vi "BiopsyBatch.vi"() -> ()   [LabVIEW 2022 SP3]
uses:
  <vilib>/Utility/file.llb/Read From Spreadsheet File (DBL).vi
  <vilib>/Analysis/NI_AALBase.lvlib
  <vilib>/Analysis/baseanly.llb/Mean (DBL).vi
panel:
  out "inc x (mm)":dbl format="%.3f"
  out "inc y (mm)":dbl format="%.3f"
  in  "Correct Data?":bool
  in  "RF pts in line":i32=110
  in  "fix rf pts?":bool=TRUE
  in  "Batch file source":u16(ring) items=["Single eye file", "All files in chosen directory", "Choose directroy and file list"]
  out "Current File":string
  in  "Choose Directory of EYE files":path=path "C:/WINDOWS/DESKTOP/rri.eye"
  out "single case fit data":T1 {"pts in fit" format="%.2f"; "midband fit" format="%.2f"; "intercept (b)" format="%.2f"; "slope (m)" format="%.3f"}
  in  "which cursors?":bool
  out "polar axis":cluster{"r axis":dbl[], "theta axis":dbl[]} {"theta axis" format="%.2f"; "r axis" format="%.2f"}
  in  "Log scaling?":bool=TRUE
  out "raw x coord":dbl[][](array[numeric]) format="%.2f"
  out "raw y coord":dbl[][](array[numeric]) format="%.2f"
  out "raw sector image":dbl[][](array[numeric]) format="%.2f"
  out "Axis scaling Params":T2 {"Y high" format="%.2f"; "Y low" format="%.2f"; "X left" format="%.2f"; "X right" format="%.2f"}
  out "Sector as data array":dbl[][](graph)
  in  "Last sector file":path
  in  "View Header?":bool
  in  "Save to Spectra.txt?":bool
  out "Cal File Att":string
  out "RF File Att":string
  in  "FFT size for":u16(ring)=6 items=["next 2^n", "8", "16", "32", "64", "128", "256", "512"]
  in  "Cal File Selection":u16(ring)=1 items=["Don't subtract a Cal File", "Use Info in Header", "Specify Cal Info"]
  in  "Cal File Name":string
  out "actual length\nof padded ROI":i32
  out "need this # of RF pts\nto match Cal File":i32
  in  "Fit band":T3={"start"=3.5, "stop freq"=8.0, "center freq"=5.75} {"center freq" format="%.2f"; "stop freq" format="%.2f"; "start" format="%.2f"}
  out "Spectrum (dBr vs. MHz)":T4(graph)
  out "Raw data":i16[][](graph)
  in  "new eye file path":path
  # "Define endpoints of biopsy ROI. Normally only need to define green and red cursor. Green lower left, red upper left, yellow lower right. Default values are those used in MSKCC study. ROI must be set up with data having 8 mm delay. Run program, then choose a file with 8 mm delay when prompted. Program can then be run again in batch mode by selecting Save to Spectra.txt. Batch operation is done on a whole directory or a list of files. Batch mode will adjust ROI to account for any cases that do not have an 8 mm delay."
  # "Spectrum Fit Parameters"
  # "Only top and bottom of sector box is shown. Ends\nmay not stop at the same scan line."
  # "© 2000-2002 Riverside Research Institute"
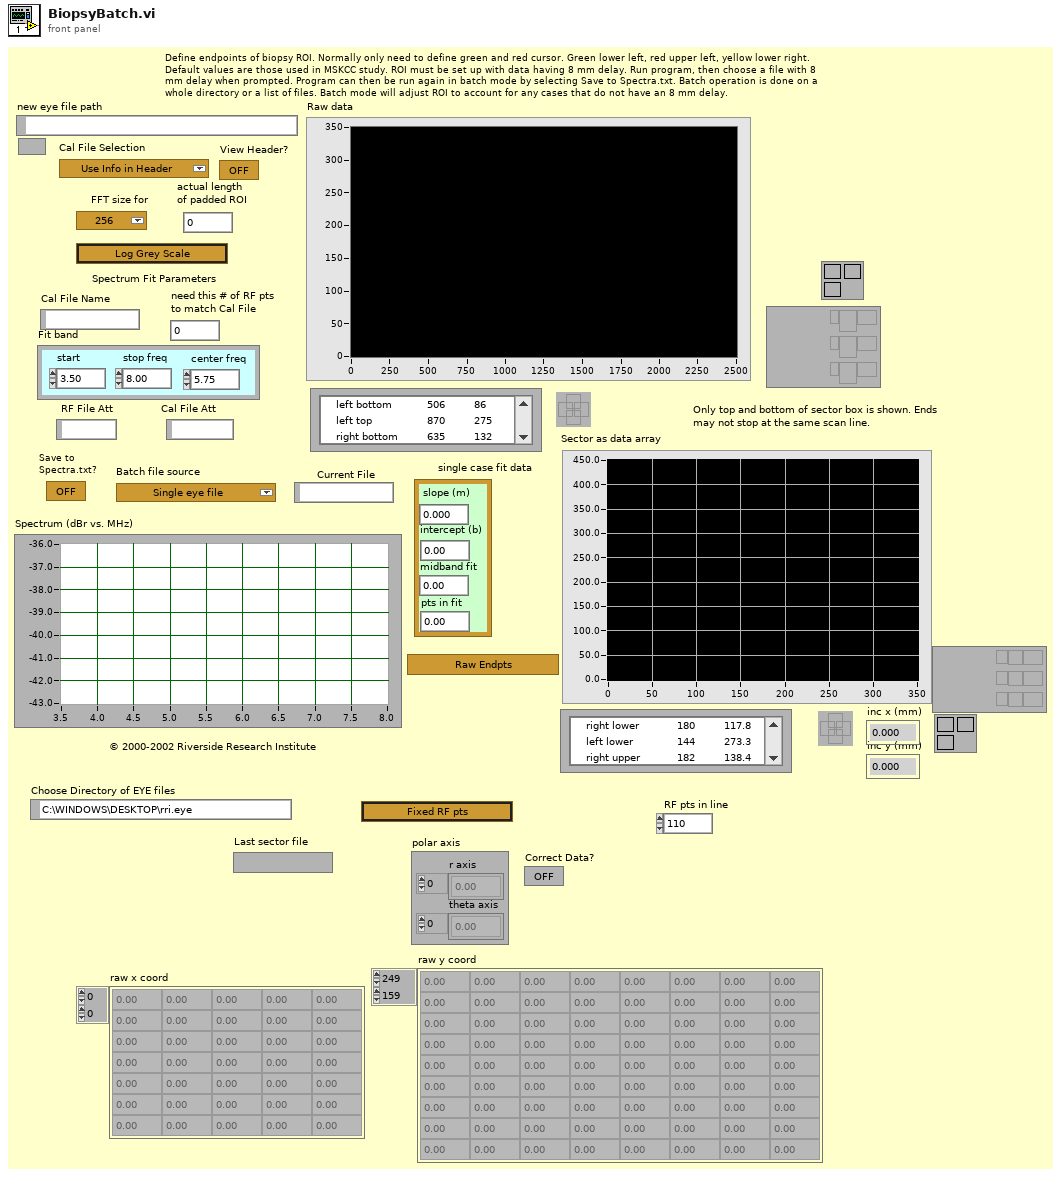
[diagram p1: front panel]
types:
  T1 = cluster{"slope (m)":dbl, "intercept (b)":dbl, "midband fit":dbl, "pts in fit":dbl}
  T2 = cluster{"X right":dbl, "X left":dbl, "Y low":dbl, "Y high":dbl}
  T3 = cluster{"start":dbl, "stop freq":dbl, "center freq":dbl}
  T4 = cluster{"fo of fit":dbl, "df (MHz)":dbl, "Best Linear Fit":dbl[]}[]
  T5 = typedef "Header.ctl" = cluster{"header info":cluster{"Header":string, "Head length":i16}, "A/D info":cluster{"# rf points per line":u16, "# lines per scan":u16, "sample rate MHz":u16, "# A/D bits":i16, "# bytes per A/D":u16, "TGC Flag":u16, "A/D Type":string}, "Tranducer Info":cluster{"bandwidth":sgl, "center freq":sgl, "start freq":sgl, "ID":i32}, "Scan Info":cluster{"delay":sgl, "pivot distance":sgl, "sector scan angle":sgl, "operator":string, "Scan Mode":string, "location":string}, "Time/Date Info":cluster{"date":string, "time":string}, "RF Info":cluster{"RF file name":string, "RF file att":string, "RF cal file name":string, "RF cal file att":string}, "Patient Info":cluster{"ID":string, "extended ID":string, "age":u16, "sex":string, "previously\nscanned":string, "PSA":sgl, "LOS":u8, "Ethnicty 2":u8, "Race":u8}, "Tissue Type":cluster{"organ":i16, "disease type":i16, "disease location":i16, "IQ_pts":u16, "RcvBuffer":u8, "RcvFrame":u16, "IQBuff":u8, "IQFrame":u16, "IQPage":u8}, "Votage scaling":cluster{"Digitizer (dB)":sgl, "Gain (dB)":sgl, "Atten (dB)":sgl}, "Comment":string, "Misc Info":cluster{"avg num":u16, "c speed":i16, "Div By or SF zones":i16, "XMIT CHS":u8, "RCV CHS":u8, "Xmit angle":sgl}, "Therapy Parameters":cluster{"Theraputic Freq (MHz)":sgl, "Time on (s)":sgl, "Therapy amplitude (mV)":sgl, "Lines Before":u16, "Lines After":u16}, "Scan Settings":cluster{"Energy (uJ or V)":u8, "Damp (Ohm) or Fc":u8, "HP Filt (KHz)":u8, "LP Filt (MHz)":u8, "Gain (db)":u8, "prf (kHz)":sgl, "Distance between\nscan lines (um)":u16, "Distance between\nscan planes (um)":u16, "Scan line gap (um)":sgl, "Scan plane gap (um)":sgl}, "Compression Parameters":cluster{"F1 (MHz)":sgl, "F2 (MHz)":sgl, "% taper":sgl, "duration":sgl}, "Patient Info Xtra":cluster{"First Name":string, "Last Name":string, "Notes":string}, "ROI Box":u16[]}
  T6 = cluster{"delay":sgl, "pivot distance":sgl, "sector scan angle":sgl, "operator":string, "Scan Mode":string, "location":string}
  T7 = cluster{"Cursor.Cursor X":dbl, "Cursor.Cursor Y":dbl, "Cursor.Cursor X":dbl, "Cursor.Cursor Y":dbl, "Cursor.Cursor X":dbl, "Cursor.Cursor Y":dbl, i32, i32}
  T8 = enum32{"existing file", "new file", "new or existing file", "existing dir", "new dir", "new or existing dir", "existing file (use LLBs)", "new file (use LLBs)", "new or existing file (use LLBs)", "new or existing file or directory (use LLBs)"}
  T9 = cluster{"bandwidth":sgl, "center freq":sgl, "start freq":sgl, "ID":i32}
  T10 = cluster{"RF file name":string, "RF file att":string, "RF cal file name":string, "RF cal file att":string}
  T11 = cluster{"RF file name":string, "RF file att":string, "Cal File Name":string, "RF cal file att":string}
  T12 = cluster{"start freq":sgl, sgl, "center freq":sgl}
  T13 = cluster{"sample rate MHz":u16, "first row":dbl[], "Fit band":cluster{"start":dbl, "stop freq":dbl, "center freq":dbl}, "RF Info":cluster{"RF file name":string, "RF file att":string, "RF cal file name":string, "RF cal file att":string}, "2-D data array":i16[][], "delay":sgl}
  T14 = cluster{"mean":dbl, "RF pts in line":i32, "Cursor.Cursor Y":dbl, i32}
  T15 = cluster{"slope (m)":dbl[][], "intercept (b)":dbl[][], "midband fit":dbl[][], "pts in fit":dbl}
  T16 = cluster{"fo of fit":dbl, "df (MHz)":dbl, dbl[]}[]
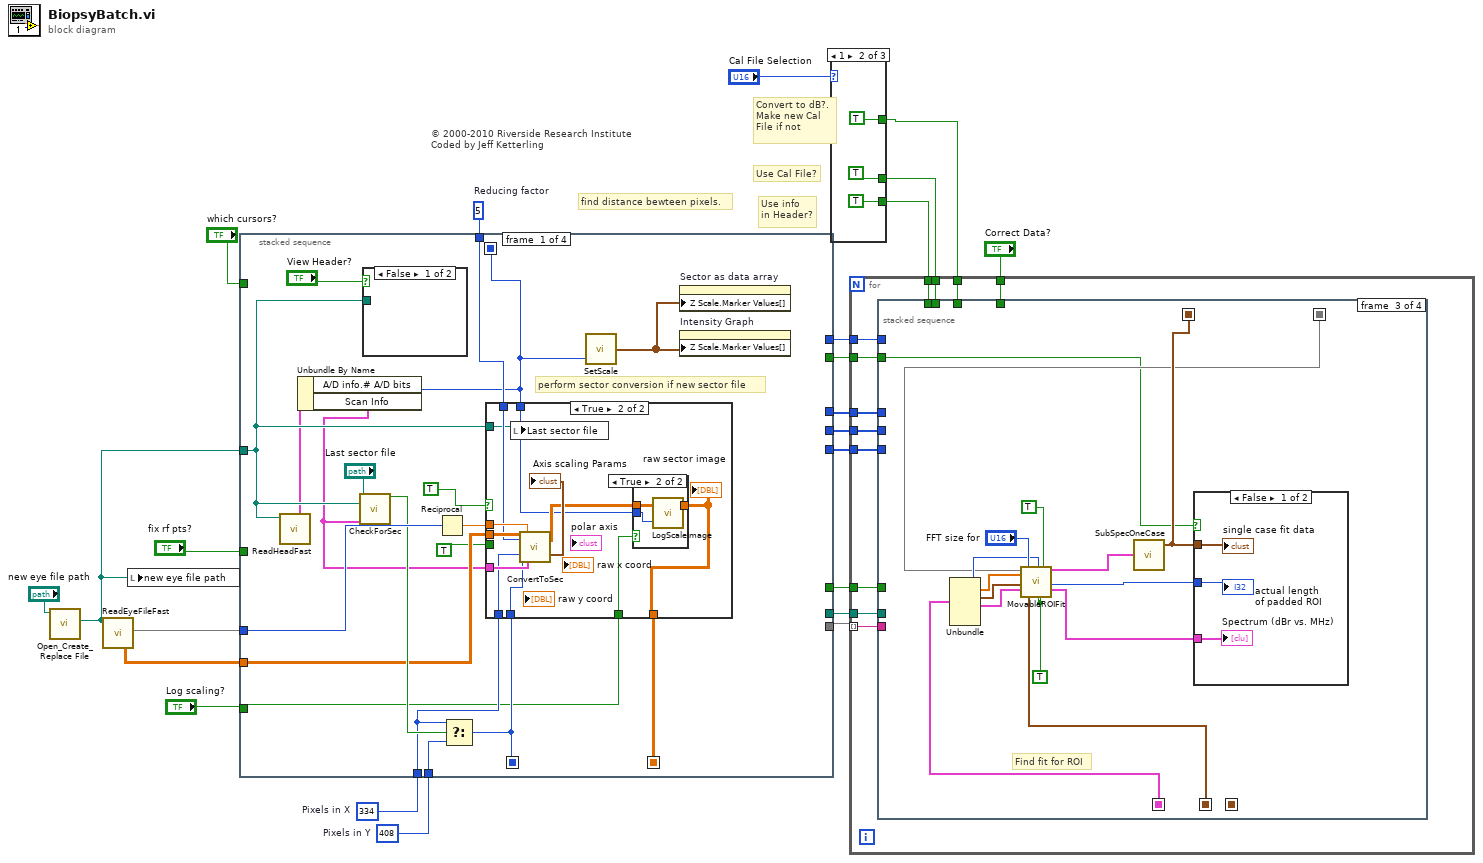
[diagram p0: block diagram]
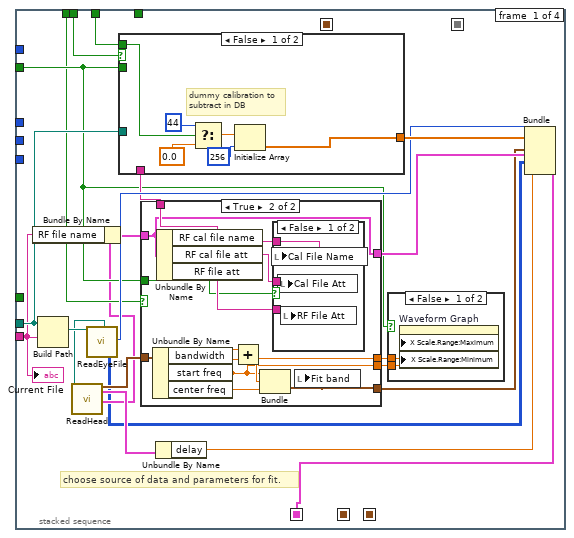
[diagram p2: hidden frame]
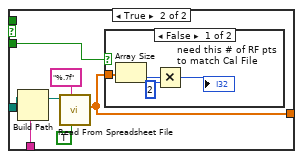
[diagram p4: hidden frame]
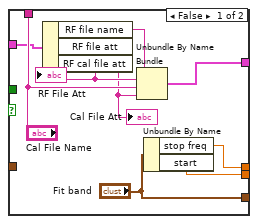
[diagram p6: hidden frame]
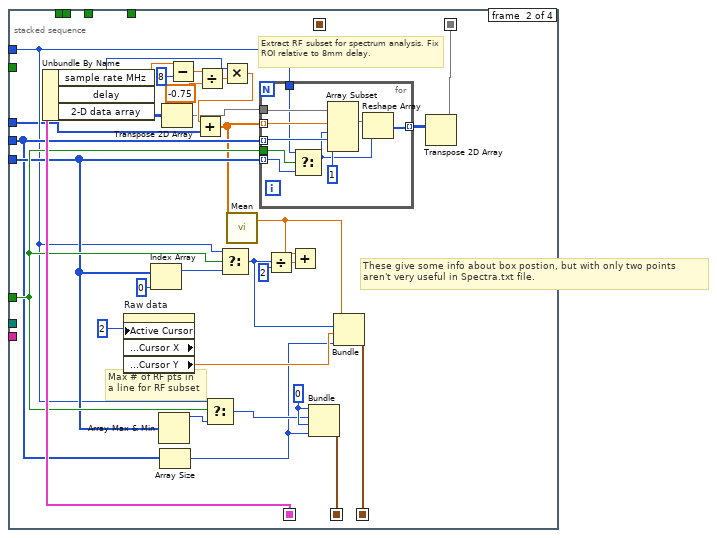
[diagram p8: hidden frame]
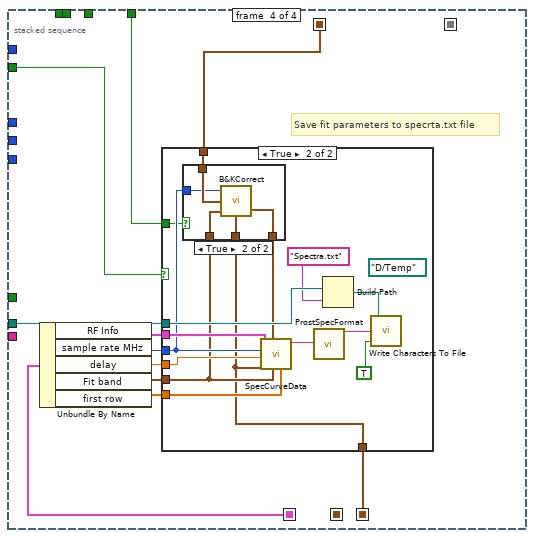
[diagram p10: hidden frame]
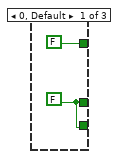
[diagram p13: hidden frame]
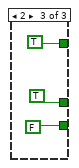
[diagram p14: hidden frame]
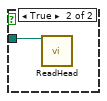
[diagram p15: hidden frame]
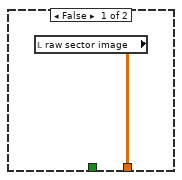
[diagram p16: hidden frame]
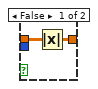
[diagram p17: hidden frame]
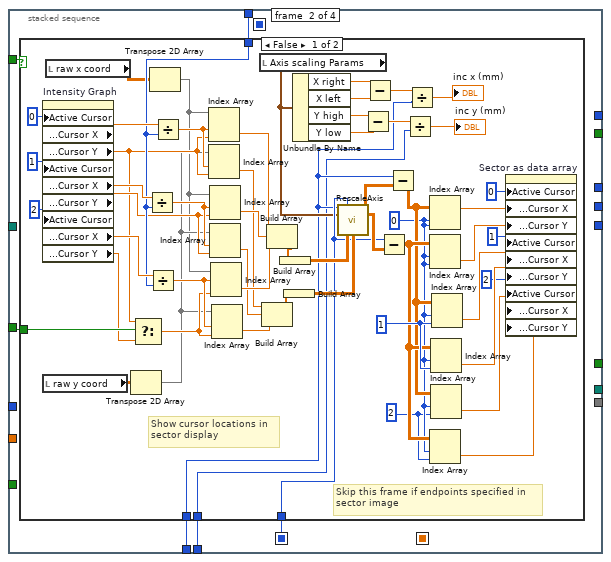
[diagram p18: hidden frame]
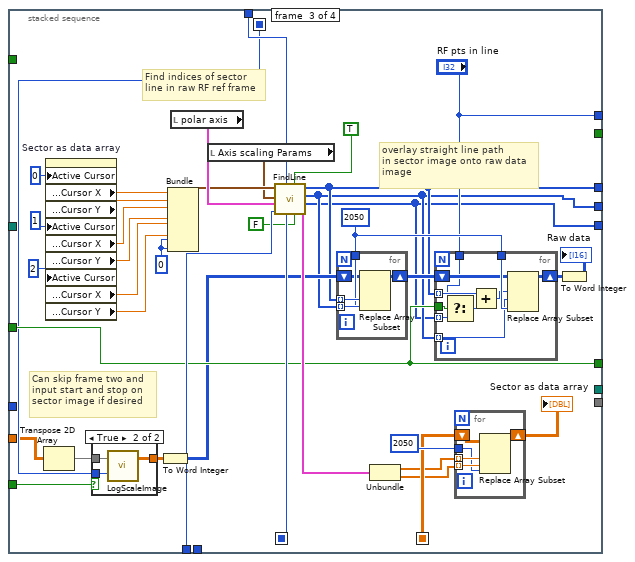
[diagram p20: hidden frame]
diagram:
  w18 = 408  # Pixels in Y
  w17 = 334  # Pixels in X
  w19 = 5  # Reducing factor
  # "find distance bewteen pixels."
  # "© 2000-2010 Riverside Research Institute\nCoded by Jeff Ketterling"
  # "Convert to dB?.\nMake new Cal\nFile if not"
  # "Use Cal File?"
  # "Use info\nin Header?"
  n1 = call <vilib>:"Open_Create_Replace File.vi"("file path"="new eye file path") -> ("new file path"=w20:path)  [unwired: 5 in, 5 out]
  n2 = call "ReadEyeFileFast.vi"("new file path"=w20) -> ("2-D data array"=w1:sgl[][], 16:w21)  [unwired: 12 in, 5 out]
  n3 = local write "new eye file path"(w20) -> ()
  n4 = stacked-sequence {
    seq-local: [w37 _ _ _] -> [_ w65 w153 _]
    seq-local: [w27 _ _ _] -> [_ _ w143 _]
    seq-local: [w26 _ _ _] -> [_ _ w134 _]
    tunnel: w21 -> [w41 _ _ _]
    tunnel: w1 -> [w33 _ w126 _]
    tunnel: w20 -> [w32 _ _ w192]
    tunnel: w19 -> [w39 w67 w159 _]
    tunnel: w18 -> [w38 w62 _ _]
    tunnel: w17 -> [w34 w66 w158 _]
    tunnel: "which cursors?" -> [_ w64 _ _]
    tunnel: [_ _ w128 _] -> w15
    tunnel: [_ _ w129 _] -> w14
    tunnel: [_ _ _ "Save to Spectra.txt?"] -> w13
    tunnel: [_ _ _ w194] -> w12
    tunnel: [_ _ _ w193] -> w11
    tunnel: [_ _ w127 _] -> w7
    tunnel: [_ _ "RF pts in line" _] -> w6
    tunnel: [_ _ w141 _] -> w5
    tunnel: "fix rf pts?" -> [_ w63 w141 _]
    tunnel: "Log scaling?" -> [w31 _ w135 _]
    frame #0 {
      # "perform sector conversion if new sector file"
      n5 = call "ReadHeadFast.vi"("new file path"=w32) -> ("Header In"=w25:T5)  [unwired: 7 in, 3 out]
      n6 = Unbundle By Name(w25) -> ("A/D info.# A/D bits"=w26:i16, "Scan Info"=w24:T6)
      n7 = call "CheckForSec.vi"("Scan Info"=w24, "Last sector file opened"=w32, "Current file"="Last sector file") -> ("= 360?"=w35:bool)  [unwired: 6 out]
      n8 = case shown="False" "View Header?" {
        tunnel: w32 -> [_ w43]
        frame False {
        }
        frame True {
          n9 = call "ReadHead.vi"("new file path"=w43) -> ()  [unwired: 19 out]
        }
      }
      n10 = Reciprocal(x=w41) -> (1/x=w42:dbl)
      n11 = Select(t=w34, s=w35, f=w38) -> (s? t:f=w37:i32)
      n12 = case shown="True" TRUE {
        tunnel: w33 -> [_ w56]
        tunnel: w24 -> [_ w55]
        tunnel: w42 -> [_ w54]
        tunnel: w39 -> [_ w52]
        tunnel: w34 -> [_ w46]
        tunnel: w37 -> [_ w45]
        tunnel: w31 -> [_ w50]
        tunnel: [w44 w49] -> w27
        tunnel: w32 -> [_ w48]
        tunnel: w26 -> [_ w47]
        tunnel: TRUE -> [_ _]
        frame False {
          n13 = local read "raw sector image"() -> (w44:dbl[][])
        }
        frame True {
          n14 = local write "Last sector file"(w48) -> ()
          n15 = call "ConvertToSec.vi"("raw image data in"=w56, "reduce pts by factor of"=w52, "pixels in x"=w46, "pixels in y"=w45, "Time between rf pts\nmicros"=w54, "Scan Info"=w55) -> ("raw sector out"=w51:dbl[][], "Axis scaling Params"=→"Axis scaling Params":T2)  [unwired: 5 in, 7 out]
          n16 = case shown="True" w50 {
            tunnel: w51 -> [w58 w61]
            tunnel: [w57 w60] -> w49
            tunnel: w47 -> [_ w59]
            frame False {
              n17 = Absolute Value(x=w58) -> (abs(x)=w57:dbl[][])
            }
            frame True {
              n18 = call "LogScaleImage.vi"("A/D bits"=w59, "input array"=w61) -> ("log scale image"=w60:dbl[][])  [unwired: 1 out]
            }
          }
          "raw sector image" <- w49
        }
      }
      n19 = call "SetScale.vi"("# A/D bits"=w26) -> ("Array"=w29:cluster{dbl, u32}[])  [unwired: 1 in]
      n20 = property on="Sector as data array" class="IntGraph (strict)"("Z Scale.Marker Values[]"=w29) -> ()  [unwired: 2 in, 2 out]
      n21 = property on="Intensity Graph" class="IntGraph (strict)"("Z Scale.Marker Values[]"=w29) -> ()  [unwired: 2 in, 2 out]
    }
    frame #1 {
      n22 = case shown="False" w64 {
        tunnel: w67 -> [w105 _]
        tunnel: w66 -> [w71 _]
        tunnel: w65 -> [w91 _]
        tunnel: w63 -> [w84 _]
        tunnel: w62 -> [w70 _]
        frame False {
          w87 = 2
          w114 = 1
          w88 = 0
          # "Skip this frame if endpoints specified in\nsector image"
          # "Show cursor locations in\nsector display"
          n23 = property on="Intensity Graph" class="IntGraph (strict)"("Active Cursor"=u32 0 ("Write Attribute"), "Active Cursor"=u32 1 ("Write Attribute"), "Active Cursor"=u32 2 ("Write Attribute")) -> ("Cursor.Cursor Position:Cursor X"=w120:dbl, "Cursor.Cursor Position:Cursor Y"=w81:dbl, "Cursor.Cursor Position:Cursor X"=w117:dbl, "Cursor.Cursor Position:Cursor Y"=w102:dbl, "Cursor.Cursor Position:Cursor X"=w106:dbl, "Cursor.Cursor Position:Cursor Y"=w83:dbl)  [unwired: 2 in, 2 out]
          n24 = local read "raw y coord"() -> (w96:dbl[][])
          n25 = local read "raw x coord"() -> (w104:dbl[][])
          n26 = Transpose 2D Array(2D array=w96) -> (transposed array=w69:dbl[][])
          n27 = Select(t=w81, s=w84, f=w83) -> (s? t:f=w82:dbl)
          n28 = Divide(x=w117, y=w105) -> (x/y=w118:dbl)
          n29 = Divide(x=w106, y=w105) -> (x/y=w103:dbl)
          n30 = Transpose 2D Array(2D array=w104) -> (transposed array=w68:dbl[][])
          n31 = Divide(x=w120, y=w105) -> (x/y=w119:dbl)
          n32 = Index Array(array=w68, index (row)=w119, index (col)=w81) -> (element=w101:dbl)
          n33 = Index Array(array=w69, index (row)=w119, index (col)=w81) -> (element=w95:dbl)
          n34 = Index Array(array=w68, index (row)=w118, index (col)=w102) -> (element=w100:dbl)
          n35 = Index Array(array=w69, index (row)=w118, index (col)=w102) -> (element=w98:dbl)
          n36 = Index Array(array=w68, index (row)=w103, index (col)=w82) -> (element=w99:dbl)
          n37 = Index Array(array=w69, index (row)=w103, index (col)=w82) -> (element=w97:dbl)
          n38 = local read "Axis scaling Params"() -> (w77:T2)
          n39 = Build Array(w95, w98, w97) -> (w121:dbl[])
          n40 = Build Array(w101, w100, w99) -> (w122:dbl[])
          n41 = Build Array(w122) -> (w94:dbl[][])
          n42 = Build Array(w121) -> (w93:dbl[][])
          n43 = Unbundle By Name(w77) -> ("X right"=w76:dbl, "X left"=w75:dbl, "Y high"=w74:dbl, "Y low"=w73:dbl)
          n44 = call "RescaleAxis.vi"("pixels in x"=w71, "pixels in y"=w91, "Axis scaling Params"=w77, "x"=w94, "y"=w93) -> ("x scaled"=w113:dbl[][], "y scaled"=w112:dbl[][])  [unwired: 9 out]
          n45 = Subtract(x=w74, y=w73) -> (x-y=w78:dbl)
          n46 = Subtract(x=w76, y=w75) -> (x-y=w72:dbl)
          n47 = Subtract(x=w91, y=w112) -> (x-y=w90:dbl[][])
          n48 = Subtract(x=w71, y=w113) -> (x-y=w89:dbl[][])
          n49 = Divide(x=w78, y=w70) -> (x/y=→"inc y (mm)":dbl)
          n50 = Divide(x=w72, y=w71) -> (x/y=→"inc x (mm)":dbl)
          n51 = Index Array(array=w89, index (row)=w88, index (col)=w88) -> (element=w111:dbl)
          n52 = Index Array(array=w90, index (row)=w88, index (col)=w88) -> (element=w110:dbl)
          n53 = Index Array(array=w90, index (row)=w88, index (col)=w87) -> (element=w85:dbl)
          n54 = Index Array(array=w90, index (row)=w88, index (col)=w114) -> (element=w108:dbl)
          n55 = Index Array(array=w89, index (row)=w88, index (col)=w87) -> (element=w86:dbl)
          n56 = Index Array(array=w89, index (row)=w88, index (col)=w114) -> (element=w109:dbl)
          n57 = property on="Sector as data array" class="IntGraph (strict)"("Active Cursor"=u32 0 ("Write Attribute"), "Cursor.Cursor Position:Cursor X"=w111, "Cursor.Cursor Position:Cursor Y"=w110, "Active Cursor"=u32 1 ("Write Attribute"), "Cursor.Cursor Position:Cursor X"=w109, "Cursor.Cursor Position:Cursor Y"=w108, "Active Cursor"=u32 2 ("Write Attribute"), "Cursor.Cursor Position:Cursor X"=w86, "Cursor.Cursor Position:Cursor Y"=w85) -> ()  [unwired: 2 in, 2 out]
        }
        frame True {
        }
      }
    }
    frame #2 {
      w133 = 0
      w149 = 2050
      # "Find indices of sector\nline in raw RF ref frame"
      # "Can skip frame two and\ninput start and stop on\nsector image if desired"
      # "overlay straight line path \nin sector image onto raw data\nimage"
      n58 = Transpose 2D Array(2D array=w126) -> (transposed array=w125:sgl[][])
      n59 = property on="Sector as data array" class="IntGraph (strict)"("Active Cursor"=u32 0 ("Write Attribute"), "Active Cursor"=u32 1 ("Write Attribute"), "Active Cursor"=u32 2 ("Write Attribute")) -> ("Cursor.Cursor Position:Cursor X"=w156:dbl, "Cursor.Cursor Position:Cursor Y"=w140:dbl, "Cursor.Cursor Position:Cursor X"=w157:dbl, "Cursor.Cursor Position:Cursor Y"=w161:dbl, "Cursor.Cursor Position:Cursor X"=w147:dbl, "Cursor.Cursor Position:Cursor Y"=w139:dbl)  [unwired: 2 in, 2 out]
      n60 = case shown="True" w135 {
        tunnel: w125 -> [w164 w168]
        tunnel: [w165 w167] -> w137
        tunnel: w134 -> [_ w166]
        frame False {
          n61 = Absolute Value(x=w164) -> (abs(x)=w165:sgl[][])
        }
        frame True {
          n62 = call "LogScaleImage.vi"("A/D bits"=w166, "input array"=w168) -> ("log scale image"=w167:dbl[][])  [unwired: 1 out]
        }
      }
      n63 = To Word Integer(number=w137) -> (16bit integer=w136:i16[][])
      n64 = Bundle("Cursor.Cursor X"=w156, "Cursor.Cursor Y"=w140, "Cursor.Cursor X"=w157, "Cursor.Cursor Y"=w161, "Cursor.Cursor X"=w147, "Cursor.Cursor Y"=w139, w133, w133) -> (w155:T7)  [unwired: 1 out]
      n65 = local read "polar axis"() -> (w160:cluster{"r axis":dbl[], "theta axis":dbl[]})
      n66 = local read "Axis scaling Params"() -> (w154:T2)
      n67 = call "FindLine.vi"("flip interp?"=FALSE, "Box?"=TRUE, "pixels in y"=w153, "reduce pts by factor of"=w159, "pixels in x"=w158, "polar axis"=w160, "Axis scaling Params"=w154, "Sector EndPts"=w155) -> ("sector image line indices"=w146:cluster{"x indices":dbl[], "y indices":dbl[]}, "length"=w127:i32[], "y indices"=w128:i32[], "x indices"=w129:i32[])
      n68 = for {
        tunnel: w149 -> [w186]
        tunnel: w129 -> [w188] mode=indexing
        tunnel: w128 -> [w187] mode=indexing
        shift-right: [w184] -> w150
        shift-left: w136 -> [w185]
        n69 = Replace Array Subset(array=w185, new element=w186, index (row)=w188, index (col)=w187) -> (w184:i16[][])
      }
      n70 = Unbundle(w146) -> ("x indices"=w131:dbl[], "y indices"=w132:dbl[])
      n71 = for {
        tunnel: w149 -> [w183]
        shift-right: [w181] -> w148
        shift-left: w150 -> [w182]
        tunnel: w128 -> [w180] mode=indexing
        tunnel: w129 -> [w178] mode=indexing
        tunnel: w127 -> [w177] mode=indexing
        tunnel: "RF pts in line" -> [w175]
        tunnel: w141 -> [w174]
        n72 = Select(t=w175, s=w174, f=w177) -> (s? t:f=w176:i32)
        n73 = Add(x=w178, y=w176) -> (x+y=w179:i32)
        n74 = Replace Array Subset(array=w182, new element=w183, index (row)=w179, index (col)=w180) -> (w181:i16[][])
      }
      n75 = for {
        tunnel: w131 -> [w173] mode=indexing
        tunnel: w132 -> [w172] mode=indexing
        shift-right: [w171] -> w145
        shift-left: w143 -> [w170]
        tunnel: 2050 -> [w169]
        n76 = Replace Array Subset(array=w170, new element=w169, index (row)=w173, index (col)=w172) -> (w171:dbl[][])
      }
      "Sector as data array" <- w145
      n77 = To Word Integer(number=w148) -> (16bit integer=→"Raw data":i16[][])
    }
    frame #3 {
      n78 = Equal To 0?(x="Batch file source") -> (x = 0?=w190:bool)
      n79 = case shown="False" w190 {
        tunnel: [w199 w213] -> w194
        tunnel: [w198 w215] -> w193
        tunnel: w192 -> [_ w216]
        tunnel: "Batch file source" -> [w195 _]
        frame False {
          (unwired) T8."existing dir" ("select mode (2)")
          # "List files from\nselected directory\nand then display the ones selected."
          n80 = Decrement(x=w195) -> (x-1=w196:u16)
          n81 = File Dialog(7:"Select Directory With EYE Files " ("prompt"), 11:"Choose Directory of EYE files") -> (3:w198:path)  [unwired: 1 in, 7 out]
          n82 = case shown="1" w196 {
            tunnel: [w202 w206] -> w199
            tunnel: w198 -> [w201 _]
            frame 0, Default {
              n83 = List Folder(path=w201, pattern="*.eye") -> (filenames=w202:string[])  [unwired: 1 in, 4 out]
            }
            frame 1 {
              n84 = File Dialog(7:"Choose list of EYE files" ("prompt")) -> (3:w205:path)  [unwired: 1 in, 8 out]
              n85 = call <vilib>:"Read Lines From File.vi"("convert eol? (no:F)"=TRUE, "file path (dialog if empty)"=w205) -> ("line string"=w212:string)  [unwired: 1 in, 6 out]
              n86 = Spreadsheet String To Array(format string="%s", spreadsheet string=w212, array type (2D Dbl)=string[][] [] ("Array Constant")) -> (array=w207:string[][])  [unwired: 1 in]
              n87 = Index Array(array=w207, index (col)=0) -> (element=w206:string[])  [unwired: 1 in]
            }
          }
          n88 = local write "Choose Directory of EYE files"(w198) -> ()
        }
        frame True {
          # "Use this if only running single test case."
          n89 = Strip Path(path=w216) -> (stripped path=w215:path, name=w214:string)
          n90 = Build Array(w214) -> (w213:string[])
        }
      }
    }
  }
  n91 = case shown="1" "Cal File Selection" {
    tunnel: [FALSE TRUE TRUE] -> w10
    tunnel: [w217 TRUE TRUE] -> w8
    tunnel: [w217 TRUE FALSE] -> w9
    frame 0, Default {
      w217 = FALSE
    }
    frame 1 {
    }
    frame 2 {
    }
  }
  n92 = for {
    tunnel: w15 -> [w236]
    tunnel: w14 -> [w235]
    tunnel: w13 -> [w234]
    tunnel: w12 -> [w233] mode=indexing
    tunnel: w11 -> [w232]
    tunnel: w10 -> [w231]
    tunnel: w9 -> [w230]
    tunnel: w8 -> [w229]
    tunnel: w7 -> [w228]
    tunnel: w6 -> [w227]
    tunnel: w5 -> [w226]
    tunnel: "Correct Data?" -> [w225]
    n93 = stacked-sequence {
      seq-local: [_ _ w353 _] -> [_ _ _ w364]
      seq-local: [_ w330 _ _] -> [_ _ w351 _]
      seq-local: [_ w317 _ _] -> [_ _ w344 _]
      seq-local: [w239 _ _ _] -> [_ w329 w349 w363]
      seq-local: [_ w325 _ _] -> [_ _ _ w362]
      tunnel: w236 -> [_ w320 _ _]
      tunnel: w235 -> [_ w305 _ _]
      tunnel: w234 -> [w248 _ w343 w366]
      tunnel: w233 -> [w243 _ _ _]
      tunnel: w232 -> [w258 _ _ w365]
      tunnel: w231 -> [w247 _ _ _]
      tunnel: w230 -> [w246 _ _ _]
      tunnel: w229 -> [w245 _ _ _]
      tunnel: w228 -> [_ w321 _ _]
      tunnel: w227 -> [_ w319 _ _]
      tunnel: w226 -> [_ w322 _ _]
      tunnel: w225 -> [_ _ _ w361]
      frame #0 {
        # "choose source of data and parameters for fit."
        n94 = Build Path(base path=w258, name or relative path=w243) -> (appended path=w253:path)
        n95 = call "ReadEyeFile.vi"("new file path"=w253) -> ("new path out"=w237:path, "2-D data array"=w238:i16[][], "sample rate MHz"=w254:u16)  [unwired: 1 in, 15 out]
        n96 = call "ReadHead.vi"("new file path"=w237) -> ("Tranducer Info"=w252:T9, "Scan Info"=w244:T6, "RF Info"=w242:T10)  [unwired: 16 out]
        n97 = Bundle By Name(cluster=w242, "RF file name"=w243) -> (w241:T10)
        n98 = case shown="True" w246 {
          tunnel: w252 -> [_ w297]
          tunnel: w241 -> [w282 w292]
          tunnel: [w280 w292] -> w257
          tunnel: ["Fit band" w287] -> w255
          tunnel: ["Cal File Name" w293] -> w251
          tunnel: w248 -> [_ w289]
          tunnel: [w284 w294] -> w250
          tunnel: [w283 w288] -> w249
          frame False {
            # "use input data for fit and plot scaling"
            n99 = Unbundle By Name(w282) -> ("RF file name"=w281:string, "RF file att"=w279:string, "RF cal file att"=w278:string)
            "RF File Att" <- w279
            "Cal File Att" <- w278
            n100 = Bundle("RF file name"=w281, "RF file att"=w279, "Cal File Name"="Cal File Name", "RF cal file att"=w278) -> (w280:T11)  [unwired: 1 out]
            n101 = Unbundle By Name("Fit band") -> ("stop freq"=w284:dbl, "start"=w283:dbl)
          }
          frame True {
            n102 = Unbundle By Name(w297) -> ("bandwidth"=w296:sgl, "start freq"=w288:sgl, "center freq"=w295:sgl)
            n103 = Unbundle By Name(w292) -> ("RF cal file name"=w293:string, "RF cal file att"=w291:string, "RF file att"=w290:string)
            n104 = Add(x=w296, y=w288) -> (x+y=w294:sgl)
            n105 = Bundle("start freq"=w288, w294, "center freq"=w295) -> (w287:T12)  [unwired: 1 out]
            n106 = case shown="False" w289 {
              tunnel: w293 -> [w300 _]
              tunnel: w291 -> [w299 _]
              tunnel: w290 -> [w298 _]
              frame False {
                n107 = local write "Cal File Name"(w300) -> ()
                n108 = local write "Cal File Att"(w299) -> ()
                n109 = local write "RF File Att"(w298) -> ()
              }
              frame True {
              }
            }
            n110 = local write "Fit band"(w287) -> ()
          }
        }
        n111 = case shown="False" w245 {
          tunnel: [w262 w267] -> w256
          tunnel: w247 -> [w261 _]
          tunnel: w258 -> [_ w270]
          tunnel: w251 -> [_ w269]
          tunnel: w248 -> [_ w268]
          frame False {
            # "Don't subtract anything\nif making a cal file"
            # "dummy calibration to\nsubtract in DB"
            n112 = Select(t=44, s=w261, f=0.0 ("t")) -> (s? t:f=w264:dbl)
            n113 = Initialize Array(w264, 256 ("Dimension Size")) -> (w262:dbl[])
          }
          frame True {
            n114 = Build Path(base path=w270, name or relative path=w269) -> (appended path=w273:path)
            n115 = call-poly <vilib>:"Read From Spreadsheet File.vi"("transpose (no:F)"=TRUE, "format (%.3f)"="%.7f", "file path (dialog if empty)"=w273) -> ("first row"=w267:dbl[])  [unwired: 1 in, 7 out]
            n116 = case shown="False" w268 {
              tunnel: w267 -> [w274 _]
              frame False {
                n117 = Array Size(array=w274) -> (size(s)=w276:i32)
                n118 = Multiply(x=w276, y=2) -> (x*y=→"need this # of RF pts\nto match Cal File":i32)
              }
              frame True {
              }
            }
          }
        }
        n119 = Unbundle By Name(w244) -> ("delay"=w240:sgl)
        n120 = case shown="False" w248 {
          tunnel: w250 -> [w260 _]
          tunnel: w249 -> [w259 _]
          frame False {
            n121 = property on="Waveform Graph" class="WFGraph (strict)"("X Scale.Range:Maximum"=w260, "X Scale.Range:Minimum"=w259) -> ()  [unwired: 2 in, 2 out]
          }
          frame True {
          }
        }
        n122 = Bundle("sample rate MHz"=w254, "first row"=w256, "Fit band"=w255, "RF Info"=w257, "2-D data array"=w238, "delay"=w240) -> (w239:T13)  [unwired: 1 out]
        "Current File" <- w243
      }
      frame #1 {
        w331 = 0
        # "These give some info about box postion, but with only two points\naren't very useful in Spectra.txt file."
        # "Max # of RF pts in\na line for RF subset"
        # "Extract RF subset for spectrum analysis. Fix ROI relative to 8mm delay."
        n123 = Unbundle By Name(w329) -> ("sample rate MHz"=w306:u16, "delay"=w307:sgl, "2-D data array"=w328:i16[][])
        n124 = property on="Raw data" class="IntGraph (strict)" props=["Active Cursor", "Cursor", "Cursor Position:Cursor X", "Cursor", "Cursor Position:Cursor Y"]("Active Cursor"=u32 2 ("Write Attribute")) -> ("Cursor.Cursor Position:Cursor Y"=w316:dbl)  [unwired: 2 in, 3 out]
        n125 = Index Array(array=w321, index=0) -> (element=w323:i32)
        n126 = Array Max & Min(array=w321) -> (max value=w318:i32)  [unwired: 3 out]
        n127 = Array Size(array=w320) -> (size(s)=w315:i32)
        n128 = Transpose 2D Array(2D array=w328) -> (transposed array=w301:i16[][])
        n129 = Subtract(x=w307, y=8) -> (x-y=w310:sgl)
        n130 = Divide(x=w310, y=-0.75) -> (x/y=w311:dbl)
        n131 = Select(t=w319, s=w322, f=w318) -> (s? t:f=w324:i32)
        n132 = Select(t=w319, s=w322, f=w323) -> (s? t:f=w312:i32)
        n133 = Multiply(x=w306, y=w311) -> (x*y=w303:dbl)
        n134 = Add(x=w303, y=w305) -> (x+y=w304:dbl[])
        n135 = call-poly <vilib>:"Mean.vi"("X"=w304) -> ("mean"=w302:dbl)  [unwired: 1 out]
        n136 = for {
          tunnel: w320 -> [w338] mode=indexing
          tunnel: w301 -> [w342]
          tunnel: [w339] -> w332 mode=indexing
          tunnel: w304 -> [w337] mode=indexing
          tunnel: w321 -> [w335] mode=indexing
          tunnel: w322 -> [w336]
          tunnel: w319 -> [w333]
          n137 = Select(t=w333, s=w336, f=w335) -> (s? t:f=w334:i32)
          n138 = Array Subset(array=w342, index (row)=w337, length (row)=w334, index (col)=w338, length (col)=1) -> (w340:i16[][])
          n139 = Reshape Array(w340, w334) -> (w339:i16[])
        }
        n140 = Divide(x=w312, y=2) -> (x/y=w313:dbl)
        n141 = Add(x=w302, y=w313) -> ()  [unwired: 1 out]
        n142 = Bundle(w331, "RF pts in line"=w324, w331, w315) -> (w330:cluster{i32, "RF pts in line":i32, i32, i32})  [unwired: 1 out]
        n143 = Bundle("mean"=w302, "RF pts in line"=w312, "Cursor.Cursor Y"=w316, w315) -> (w325:T14)  [unwired: 1 out]
        n144 = Transpose 2D Array(2D array=w332) -> (transposed array=w317:i16[][])
      }
      frame #2 {
        w356 = TRUE
        # "Find fit for ROI"
        n145 = Unbundle(w349) -> ("sample rate MHz"=w348:u16, "first row"=w347:dbl[], "Fit band"=w346:T3, "RF Info"=w345:T10)  [unwired: 2 out]
        n146 = call "MovableROIFit.vi"("input array"=w344, "calibration data"=w347, "Fit band"=w346, "RF Info"=w345, "FFT size for"="FFT size for", "Fit array"=w351, "freq (MHz)"=w348, "Single ROI?"=w356, "subtract spectrum\nfrom fit?"=TRUE, "convert output to dB?"=w356) -> ("Raw Fit Data"=w354:T15, "Length of padded array"=w350:i32, "Plots"=w357:T16)  [unwired: 3 in, 4 out]
        n147 = call "SubSpecOneCase.vi"("Raw Fit Data"=w354) -> ("single case fit data"=w353:T1)  [unwired: 3 in, 5 out]
        n148 = case shown="False" w343 {
          tunnel: w357 -> [w360 _]
          tunnel: w353 -> [w359 _]
          tunnel: w350 -> [w358 _]
          frame False {
            "Spectrum (dBr vs. MHz)" <- w360
            "single case fit data" <- w359
            "actual length\nof padded ROI" <- w358
          }
          frame True {
          }
        }
      }
      frame #3 {
        # "Save fit parameters to specrta.txt file"
        n149 = Unbundle By Name(w363) -> ("RF Info"=w367:T10, "sample rate MHz"=w368:u16, "delay"=w369:sgl, "Fit band"=w370:T3, "first row"=w371:dbl[])
        n150 = case shown="True" w366 {
          tunnel: w364 -> [_ w377]
          tunnel: w362 -> [_ w373]
          tunnel: w371 -> [_ w385]
          tunnel: w370 -> [_ w374]
          tunnel: w369 -> [_ w384]
          tunnel: w367 -> [_ w383]
          tunnel: w365 -> [_ w380]
          tunnel: w368 -> [_ w375]
          tunnel: w361 -> [_ w372]
          frame False {
          }
          frame True {
            (unwired) path "D:/Temp"
            n151 = case shown="True" w372 {
              tunnel: w377 -> [w387 w392]
              tunnel: [w387 w391] -> w376
              tunnel: w375 -> [_ w390]
              tunnel: w374 -> [_ w389]
              tunnel: w373 -> [_ w388]
              frame False {
              }
              frame True {
                n152 = call "B&KCorrect.vi"("sample rate MHz"=w390, "Fit params"=w392, "Fit band"=w389, "Array Subset"=w388) -> ("Fit params Corrected"=w391:T1)  [unwired: 2 in]
              }
            }
            n153 = call "SpecCurveData.vi"("spectal data"=w385, "Fit band"=w374, "Fit params"=w376, "Array Subset"=w373, "delay"=w384, "sample rate MHz"=w375, "RF Info"=w383) -> ("Spectra data"=w382:string)  [unwired: 4 out]
            n154 = call "ProstSpecFormat.vi"("Spectra.txt old (string)"=w382) -> ("Spectra.txt new out"=w381:string)
            n155 = Build Path(base path=w380, name or relative path="Spectra.txt") -> (appended path=w378:path)
            n156 = call <vilib>:"Write Characters To File.vi"("append to file? (new file:F)"=TRUE, "character string"=w381, "file path (dialog if empty)"=w378) -> ()  [unwired: 3 out]
          }
        }
      }
    }
  }
